vi "act-0010-2-cor.vi"() -> ()   [LabVIEW 2010]
uses:
  lv_01/lv_01.lvlib
panel:
  out "affichage":dbl caption="Temp simulée en °F"
  in  "sélecteur":bool
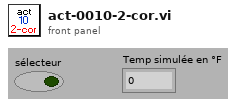
[diagram p1: front panel]
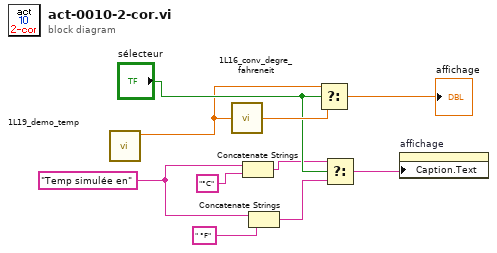
[diagram p0: block diagram]
diagram:
  w6 = "Temp simulée en"
  n1 = call "1L19_demo_temp.vi"() -> ("temp"=w3:dbl)  [unwired: 6 in, 1 out]
  n2 = call "1L16_conv_degre_fahreneit.vi"("Deg C"=w3) -> ("Deg F"=w10:dbl)
  n3 = Concatenate Strings(w6, "°C" ("Étiquette.Texte")) -> (w4:string)
  n4 = Concatenate Strings(w6, " °F" ("Étiquette.Texte")) -> (w2:string)
  n5 = Select(t=w3, s="sélecteur", f=w10) -> (s? t:f=→"affichage":dbl)
  n6 = Select(t=w4, s="sélecteur", f=w2) -> (s? t:f=w1:string)
  n7 = property on="affichage" class="NumDig (strict)"("Caption.Text"=w1) -> ()  [unwired: 2 in, 2 out]
